vi "New Network Interface.vi"(7 "Log Alias":string, 8 "Log Instance":refnum<class "LoggerReference.lvclass">, 9 "Max Number of Connections to Create (1)":i32=1, 10 "MessageProtocol":refnum<class "IMessagingProtocol.lvclass">, 11 "Connection Factory Type":refnum<class "IConnectionFactory.lvclass">) -> (0 "error out":errorcluster, 3 "Network Interface Reference":refnum<data-value>)   [LabVIEW 2017, in "Network Interface.lvlib" / "Network Interface.lvclass"]
uses:
  <vilib>/gpm_packages/@cs/Network-sink/Source/Network Interface/Network Interface/Network Interface.lvclass
  <vilib>/gpm_packages/@cs/Network-sink/Source/Network Interface/IConnectionFactory/IConnectionFactory.lvclass
  <vilib>/gpm_packages/@cs/Network-sink/Source/Network Interface/IMessagingProtocol/IMessagingProtocol.lvclass
  <vilib>/gpm_packages/@cs/event-logger/Source/Composed Log/LoggerReference/LoggerReference.lvclass
  <vilib>/gpm_packages/@cs/Network-sink/Source/Network Interface/Network Interface/Network Interface.lvclass/Network Interface.ctl
  <vilib>/gpm_packages/@cs/Network-sink/Source/Network Interface/Network Session Handler/Network Session Handler.lvclass
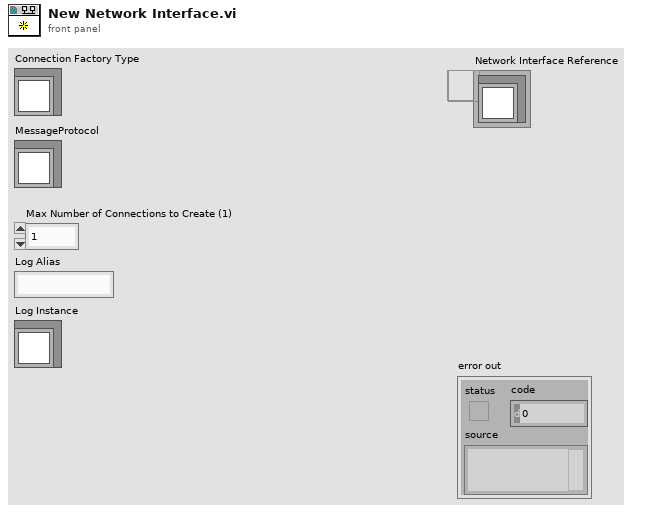
[diagram p1: front panel]
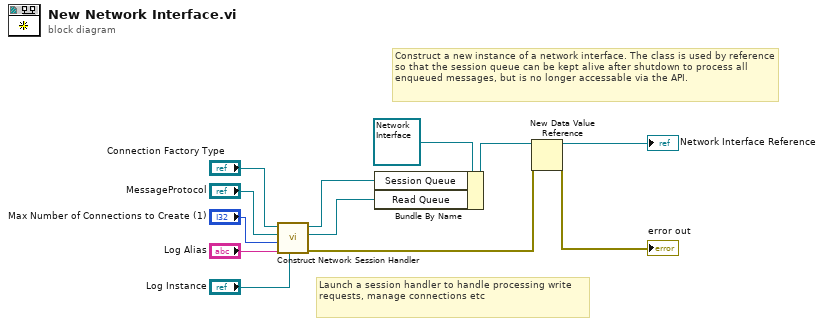
[diagram p0: block diagram]
diagram:
  # "Launch a session handler to handle processing write requests, manage connections etc"
  # "Construct a new instance of a network interface. The class is used by reference so that the session queue can be kept alive after shutdown to process all enqueued messages, but is no longer accessable via the API."
  n1 = call <vilib>:"Construct Network Session Handler.vi"("Log Instance"="Log Instance", "Log Alias"="Log Alias", "Max Number of Connections"="Max Number of Connections to Create (1)", "MessageProtocol"="MessageProtocol", "Connection Factory"="Connection Factory Type") -> ("error out"=w6:errorcluster, "Read Queue"=w7:refnum<queue>, "Session Queue"=w8:refnum<class "Message Queue.lvclass">)  [unwired: 4 in]
  n2 = Bundle By Name(cluster=refnum<class "Network Interface.lvclass"> refnum ("Network Interface in"), "Session Queue"=w8, "Read Queue"=w7) -> (w9:refnum<class "Network Interface.lvclass">)
  n3 = New Data Value Reference(data value=w9, error in=w6) -> (data value reference=→"Network Interface Reference":refnum<data-value>, error out=→"error out":errorcluster)
